vi "Button Init.vi"(8 "error in (no error)":errorcluster) -> (0 "error out":errorcluster, 3 "Buttons":T1)   [LabVIEW 2020]
uses:
  <vilib>/High Genius/HG_WSI_Tookit/Dependencies/Library/Digital Input and Output/Digital Input and Output.lvclass
  C:/Program Files (x86)/National Instruments/LabVIEW 2020/vi.lib/High Genius/HG_WSI_Tookit/Dependencies/Library/HG_LIB/HG_LIB.lvclass
  <vilib>/High Genius/HG_WSI_Tookit/Dependencies/Library/HG_LIB/HG_LIB.lvclass
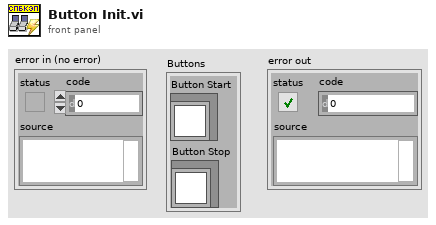
[diagram p1: front panel]
types:
  T1 = cluster{"Button Start":refnum<class "Digital Input and Output.lvclass">, "Button Stop":refnum<class "Digital Input and Output.lvclass">}
  T2 = enum16{"DI", "DO", "AI", "Pulse", "PWM", "ISQ", "ENC", "CAN", "IIC", "IMU"}
  T3 = enum16{"0", "1", "2", "3", "4", "5", "6", "7", "8", "9", "10", "11", "12", "13", "14", "15", "16", "17", "18", "19", "20", "21", "22", "23", "24", "25"}
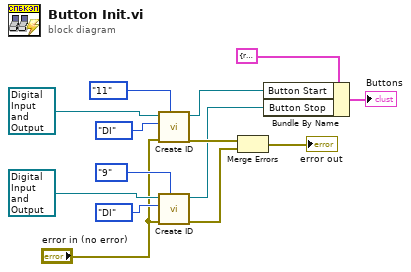
[diagram p0: block diagram]
diagram:
  n1 = call <vilib>:"Create ID.vi"("NO"=T3."11", "error in (no error)"="error in (no error)", "Function"=T2."DI", "HG_LIB in"=refnum<class "Digital Input and Output.lvclass"> refnum ("Digital Input and Output.lvclass")) -> ("error out"=w8:errorcluster, "HG_LIB out"=w2:refnum<class "Digital Input and Output.lvclass">)  [unwired: 6 in]
  n2 = call <vilib>:"Create ID.vi"("NO"=T3."9", "error in (no error)"="error in (no error)", "Function"=T2."DI", "HG_LIB in"=refnum<class "Digital Input and Output.lvclass"> refnum ("Digital Input and Output.lvclass")) -> ("error out"=w7:errorcluster, "HG_LIB out"=w1:refnum<class "Digital Input and Output.lvclass">)  [unwired: 6 in]
  n3 = Merge Errors(w8, w7) -> (→"error out":errorcluster)
  n4 = Bundle By Name(cluster=T1 {"Button Start"=refnum, "Button Stop"=refnum} ("HG_LIB out"), "Button Start"=w2, "Button Stop"=w1) -> (→"Buttons":T1)
